vi "Cmd.Reset.vi"(6 "Timeout [ms] (1000)":i32=1000, 8 "error in":errorcluster, 11 "cID in":refnum<k5>) -> (0 "error out":errorcluster, 3 "cID out":refnum<k5>)   [LabVIEW 2016]
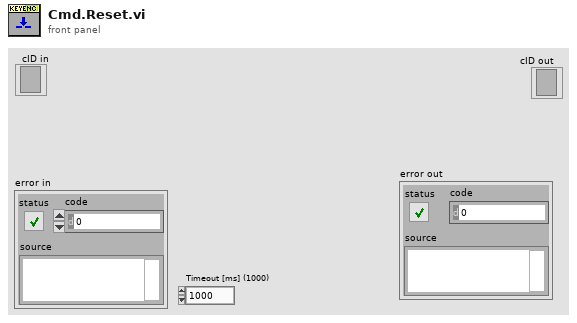
[diagram p1: front panel]
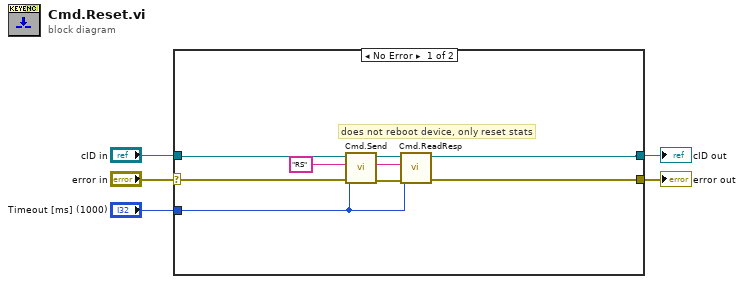
[diagram p0: block diagram]
diagram:
  n1 = case shown="No Error" "error in" {
    selector: "error in" -> [w12 w14]
    tunnel: "Timeout [ms] (1000)" -> [w9 _]
    tunnel: "cID in" -> [w13 w15]
    tunnel: [w8 w15] -> w2
    tunnel: [w7 w14] -> w1
    frame No Error {
      w6 = "RS"
      # "does not reboot device, only reset stats"
      n2 = call "Cmd.Send.vi"("error in (no error)"=w12, "Timeout [ms] (1000)"=w9, "Command"=w6, "connection ID"=w13) -> ("error out"=w10:errorcluster, "connection ID out"=w11:refnum<k5>)  [unwired: 6 in]
      n3 = call "Cmd.ReadResp.vi"("error in (no error)"=w10, "Timeout [ms] (1000)"=w9, "Request"=w6, "connection ID"=w11) -> ("error out"=w7:errorcluster, "connection ID out"=w8:refnum<k5>)  [unwired: 5 in, 1 out]
    }
    frame Error {
    }
  }
  "cID out" <- w2
  "error out" <- w1
